vi "niFPGA Linear Interpolation_m.vi"   [LabVIEW 2017]
doc: "Performs linear interpolation to approximate a function evaluation at an arbitrary location in an interval between two known points. The data type you wire to <B>y0</B> determines the output <B>y</B> data type."
uses:
  <vilib>/rvi/Analysis/common/FxpNativeNode/niFpgaFxpNative.xnode
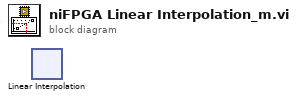
[diagram p0: block diagram]
diagram:
  n1 = xnode ("Linear Interpolation")() -> ()  [unwired: 3 in, 1 out]
